vi "Filter VIs by Name Prefix.vi"(10 "regular expression":string, 11 "Array in":path[](array[path])) -> (3 "Array out":path[](array[path]))   [LabVIEW 2020, in "Coverage Analyzer.lvlib" / "Coverage Analyzer.lvclass"]
uses:
  Coverage Analyzer.lvclass
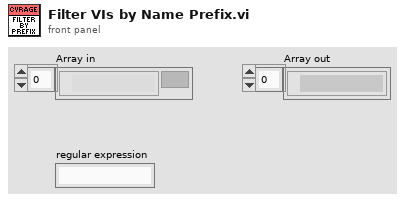
[diagram p1: front panel]
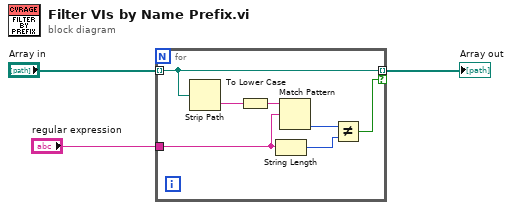
[diagram p0: block diagram]
diagram:
  n1 = for {
    tunnel: [w7] -> w2 mode=indexing if=w8
    tunnel: "Array in" -> [w7] mode=indexing
    tunnel: "regular expression" -> [w4]
    n2 = Strip Path(path=w7) -> (name=w6:string)  [unwired: 1 out]
    n3 = To Lower Case(string=w6) -> (all lower case string=w10:string)
    n4 = String Length(string=w4) -> (length=w5:i32)
    n5 = Match Pattern(string=w10, regular expression=w4) -> (offset past match=w9:i32)  [unwired: 1 in, 3 out]
    n6 = Not Equal?(x=w9, y=w5) -> (x != y?=w8:bool)
  }
  "Array out" <- w2
